vi "Read.vi"(8 "error in (no error)":errorcluster, 9 "Variant":variant, 11 "RS232 to GPIB ConvBox in":refnum<class "RSxxx to GPIB ConvBox.lvclass">) -> (0 "error out":errorcluster, 2 "String":string, 3 "RS232 to GPIB ConvBox out":refnum<class "RSxxx to GPIB ConvBox.lvclass">)   [LabVIEW 2019, in "Protocols.lvlib" / "RSxxx to GPIB ConvBox.lvclass"]
uses:
  RSxxx to GPIB ConvBox.lvclass
  Protocol Parent/Methods/Read Parameter.ctl
  RSxxx to GPIB ConvBox.lvclass/RSxxx to GPIB ConvBox.ctl
  Data Access/Read Port Ref.vi
  Data Access/Read GPIB Address.vi
  Data Access/Write Port Ref.vi
  <vilib>/dlg_ctls.llb/Space Constant.vi
  SubVIs/Status ConvBox.vi
  SubVIs/CheckListener ConvBox.vi
  <vilib>/Utility/error.llb/Clear Errors.vi
  <vilib>/Utility/error.llb/Error Cluster From Error Code.vi
  Protocol Parent/Protocol Parent.lvclass
  Protocols.lvlib
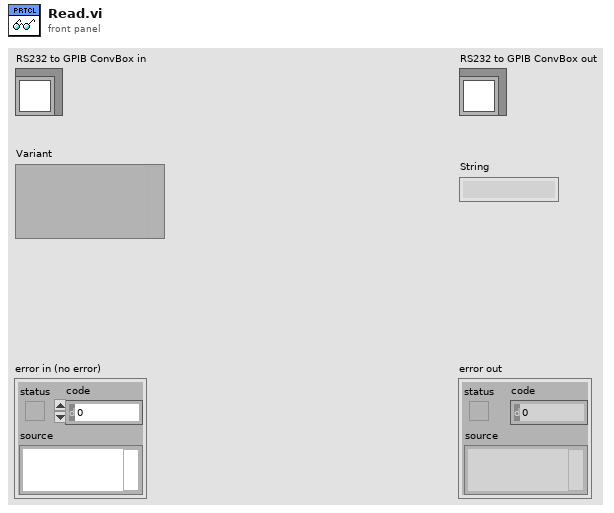
[diagram p1: front panel]
types:
  T1 = typedef "Protocols.lvlib/Protocol Parent.lvclass/Read Parameter.ctl" = cluster{"Wait Type":enum16{"Byte Count", "Wait sec"}, "Wait Value":dbl}
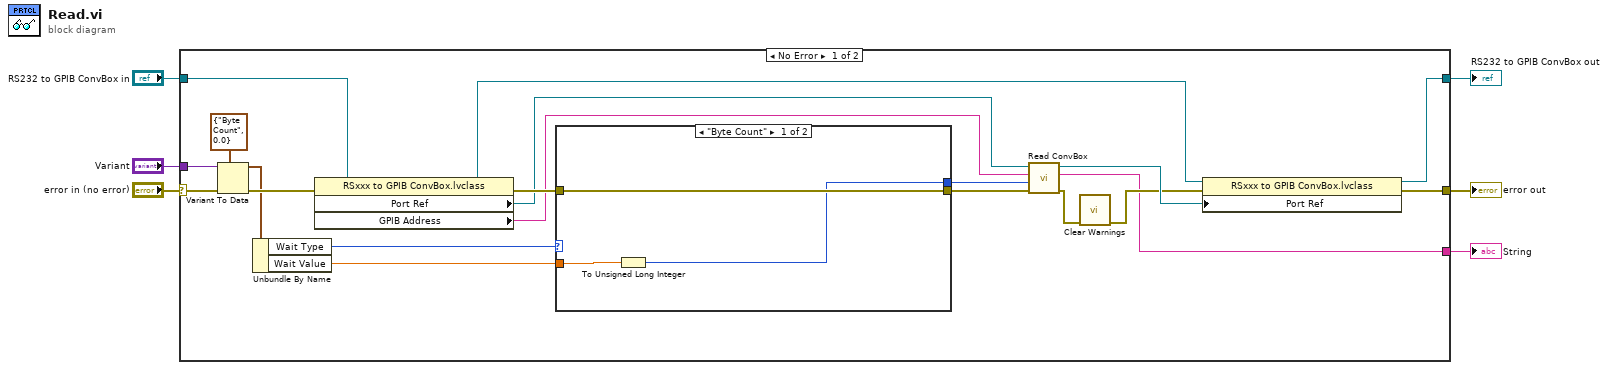
[diagram p0: block diagram]
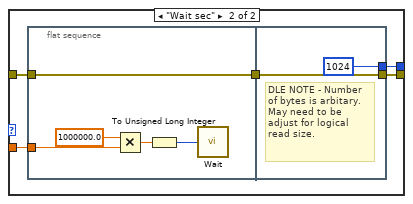
[diagram p2: hidden frame]
diagram:
  n1 = case shown="No Error" "error in (no error)" {
    selector: "error in (no error)" -> [w21 w43]
    tunnel: "RS232 to GPIB ConvBox in" -> [w26 w42]
    tunnel: [w24 w43] -> w3
    tunnel: [w22 w42] -> w2
    tunnel: "Variant" -> [w19 _]
    tunnel: [w9 _] -> w1
    frame No Error {
      n2 = Variant To Data(error in=w21, type=T1 {"Wait Type"=enum."Byte Count", "Wait Value"=0.0} ("Read Parameter"), Variant=w19) -> (data=w18:T1, error out=w20:errorcluster)
      n3 = Unbundle By Name(w18) -> ("Wait Type"=w15:enum16{"Byte Count", "Wait sec"}, "Wait Value"=w14:dbl)
      n4 = property class="RSxxx to GPIB ConvBox.lvclass"(reference=w26, error in=w20) -> (reference out=w23:refnum<class "RSxxx to GPIB ConvBox.lvclass">, error out=w17:errorcluster, "Port Ref"=w8:refnum<visa-resource-name>, "GPIB Address"=w7:string)
      n5 = case shown="\"Byte Count\"" w15 {
        tunnel: w17 -> [w29 w34]
        tunnel: [w29 w33] -> w16
        tunnel: [w27 w32] -> w10
        tunnel: w14 -> [w28 w30]
        frame "Byte Count" {
          n6 = To Unsigned Long Integer(number=w28) -> (unsigned 32bit integer=w27:u32)
        }
        frame "Wait sec" {
          n7 = flat-sequence {
            tunnel: w34 -> [w39]
            tunnel: [w39] -> w31
            tunnel: w30 -> [w36]
            tunnel: [w41] -> w33
            tunnel: [u32 1024 ("Bytes at Port")] -> w32
            tunnel: w31 -> [w41]
            frame #0 {
              n8 = Multiply(x=1000000.0, y=w36) -> (x*y=w37:dbl)
              n9 = To Unsigned Long Integer(number=w37) -> (unsigned 32bit integer=w35:u32)
              n10 = call "Wait"("Count(uSec)"=w35) -> ()  [unwired: 1 out]
            }
            frame #1 {
              # "DLE NOTE - Number of bytes is arbitary. May need to be adjust for logical read size."
            }
          }
        }
      }
      n11 = call "Read ConvBox.vi"("error in"=w16, "byte count"=w10, "address string"=w7, "VISA resource in"=w8) -> ("error out"=w12:errorcluster, "data"=w9:string, "VISA resource out"=w25:refnum<visa-resource-name>)  [unwired: 4 in, 1 out]
      n12 = call "Clear Warnings.vi"("error in (no error)"=w12) -> ("error out"=w11:errorcluster)  [unwired: 10 in]
      n13 = property class="RSxxx to GPIB ConvBox.lvclass"(reference=w23, error in=w11, "Port Ref"=w25) -> (reference out=w22:refnum<class "RSxxx to GPIB ConvBox.lvclass">, error out=w24:errorcluster)
    }
    frame Error {
    }
  }
  "error out" <- w3
  "RS232 to GPIB ConvBox out" <- w2
  "String" <- w1
